vi "FTW-ERR-StatusError.vi"(1 "error to check":errorcluster) -> (0 "Error?":bool)   [LabVIEW 2012]
panel:
  # "Inputs"
  # "Outputs"
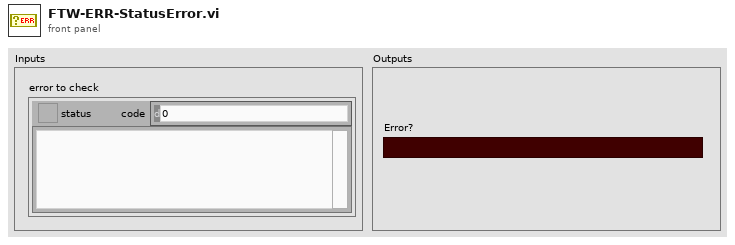
[diagram p1: front panel]
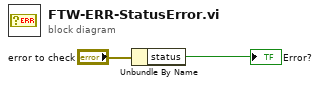
[diagram p0: block diagram]
diagram:
  n1 = Unbundle By Name("error to check") -> ("status"=→"Error?":bool)
